vi "Threshold for axis.vi"(11 "X axis":i32) -> (3 "Numeric":i32)   [LabVIEW 2015]
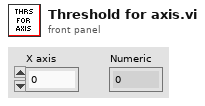
[diagram p1: front panel]
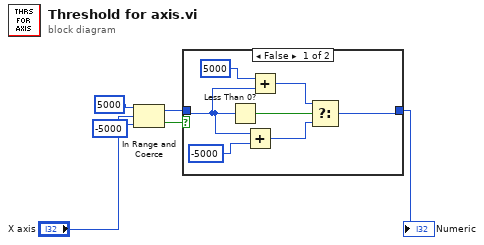
[diagram p0: block diagram]
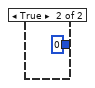
[diagram p2: hidden frame]
diagram:
  n1 = In Range and Coerce(upper limit=5000, x="X axis", lower limit=-5000 ("upper limit")) -> (coerced(x)=w5:i32, In Range?=w4:bool)
  n2 = case shown="False" w4 {
    tunnel: w5 -> [w9 _]
    tunnel: [w10 0] -> w6
    frame False {
      n3 = Less Than 0?(x=w9) -> (x < 0?=w13:bool)
      n4 = Add(x=w9, y=-5000 ("upper limit")) -> (x+y=w12:i32)
      n5 = Add(x=5000 ("upper limit"), y=w9) -> (x+y=w11:i32)
      n6 = Select(t=w11, s=w13, f=w12) -> (s? t:f=w10:i32)
    }
    frame True {
    }
  }
  "Numeric" <- w6
